vi "Create.vi"(8 "error in (no error)":errorcluster, 10 "DSP binary path":path, 11 "connection ID":i32=-1) -> (0 "error out":errorcluster, 3 "MicroDAQ.lvlib:DSP.lvclass":refnum<class "DSP.lvclass">)   [LabVIEW 2009, in "MicroDAQ.lvlib" / "DSP.lvclass"]
doc: "THis function starts DSP context and sends memory initial memory values to device."
uses:
  <instrlib>/MicroDAQ/Channel/DSP/DSP.lvclass
  <instrlib>/MicroDAQ/Channel/DSP/DSP.lvclass/DSP.ctl
  <instrlib>/MicroDAQ/Channel/Channel.lvclass
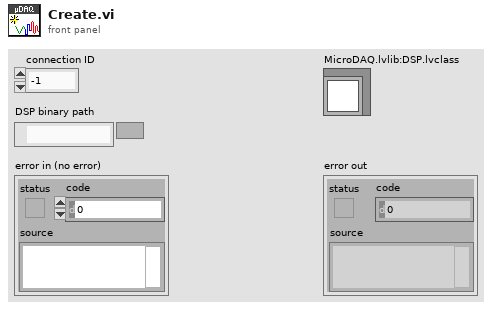
[diagram p1: front panel]
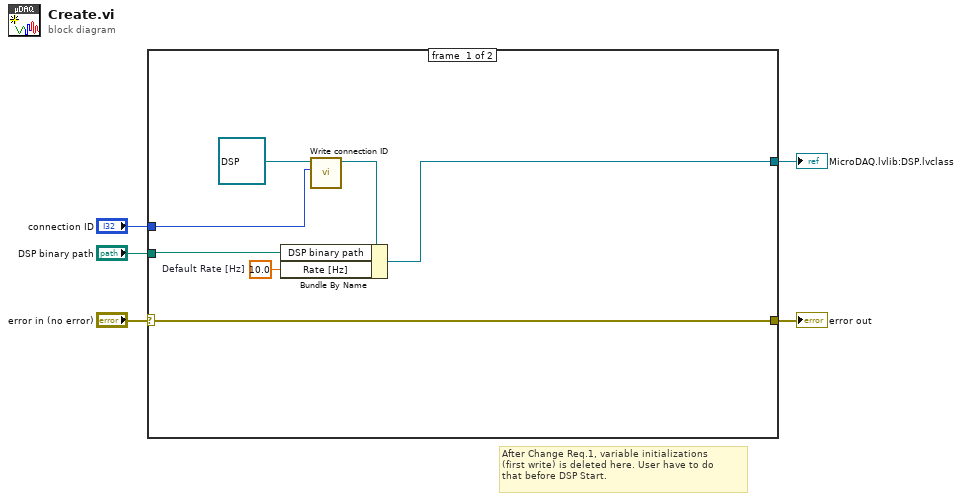
[diagram p0: block diagram]
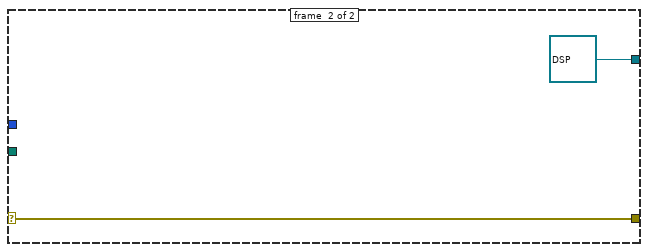
[diagram p2: hidden frame]
diagram:
  # "After Change Req.1, variable initializations\n(first write) is deleted here. User have to do\nthat before DSP Start."
  n1 = case shown="No Error" "error in (no error)" {
    selector: "error in (no error)" -> [w6 w14]
    tunnel: [w6 w14] -> w4
    tunnel: [w7 refnum<class "DSP.lvclass"> refnum ("MicroDAQ.lvlib:DSP.lvclass")] -> w3
    tunnel: "connection ID" -> [w11 _]
    tunnel: "DSP binary path" -> [w9 _]
    frame #0 {
      w8 = 10.0  # Default Rate [Hz]
      n2 = call <instrlib>:"Write connection ID.vi"("connection ID"=w11, "Task in"=refnum<class "DSP.lvclass"> refnum ("MicroDAQ.lvlib:DSP.lvclass")) -> ("Task out"=w10:refnum<class "DSP.lvclass">)  [unwired: 9 in]
      n3 = Bundle By Name(cluster=w10, "DSP binary path"=w9, "Rate [Hz]"=w8) -> (w7:refnum<class "DSP.lvclass">)
    }
    frame #1 {
    }
  }
  "error out" <- w4
  "MicroDAQ.lvlib:DSP.lvclass" <- w3
